vi "Split Single-line Reason Parts.vi"(7 "Single-line -& Reason":string) -> (4 "CSM Name":string, 8 "`State":string, 15 "`Arguments":string)   [LabVIEW 2017, in "CSM Shared.lvlib"]
uses:
  CSM Shared.lvlib
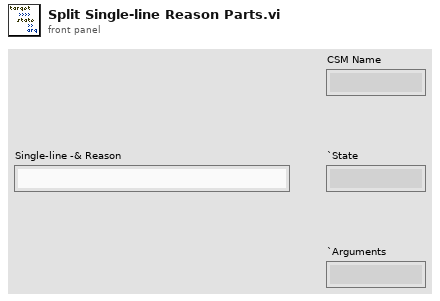
[diagram p1: front panel]
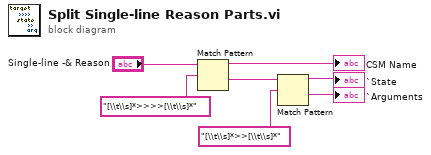
[diagram p0: block diagram]
diagram:
  n1 = Match Pattern(string="Single-line -& Reason", regular expression="[\\t\\s]*>>>>[\\t\\s]*") -> (before substring=→"CSM Name":string, after substring=w5:string)  [unwired: 1 in, 2 out]
  n2 = Match Pattern(string=w5, regular expression="[\\t\\s]*>>[\\t\\s]*") -> (before substring=→"`State":string, after substring=→"`Arguments":string)  [unwired: 1 in, 2 out]
